vi "Initialize file (SubVI).vi"(8 "error in":errorcluster) -> (0 "error out":errorcluster, 3 "Byte Stream File out":refnum<file>)   [LabVIEW 2023]
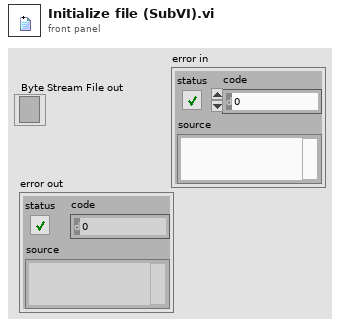
[diagram p1: front panel]
types:
  T1 = enum16{"open", "replace", "create", "open or create", "replace or create", "replace or create with confirmation"}
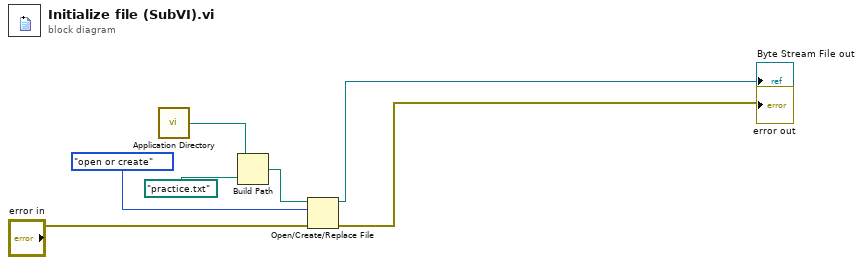
[diagram p0: block diagram]
diagram:
  n1 = call <vilib>:"Application Directory.vi"() -> ("Application Directory"=w7:path)
  n2 = Build Path(base path=w7, name or relative path=path "practice.txt") -> (appended path=w5:path)
  n3 = Open/Create/Replace File(file path (use dialog)=w5, error in="error in", operation (0:open)=T1."open or create") -> (refnum out=→"Byte Stream File out":refnum<file>, error out=→"error out":errorcluster)  [unwired: 3 in, 1 out]
